vi "motortestMeng3.vi"() -> ()   [LabVIEW 2014]
uses:
  <vilib>/Utility/inputDevices.llb/joystickAcquire.vi
  <vilib>/Utility/inputDevices.llb/closeJoystick.vi
panel:
  in  "fRelDist":sgl
  in  "MG17Motor":refnum<k7>(container)
  out "Numeric":i32
  out "pfPosition":sgl
  in  "stop 2":bool
  in  "MG17Motor 2":refnum<k7>(container)
  out "button info":T1
  out "axis info":T2
  in  "stop":bool
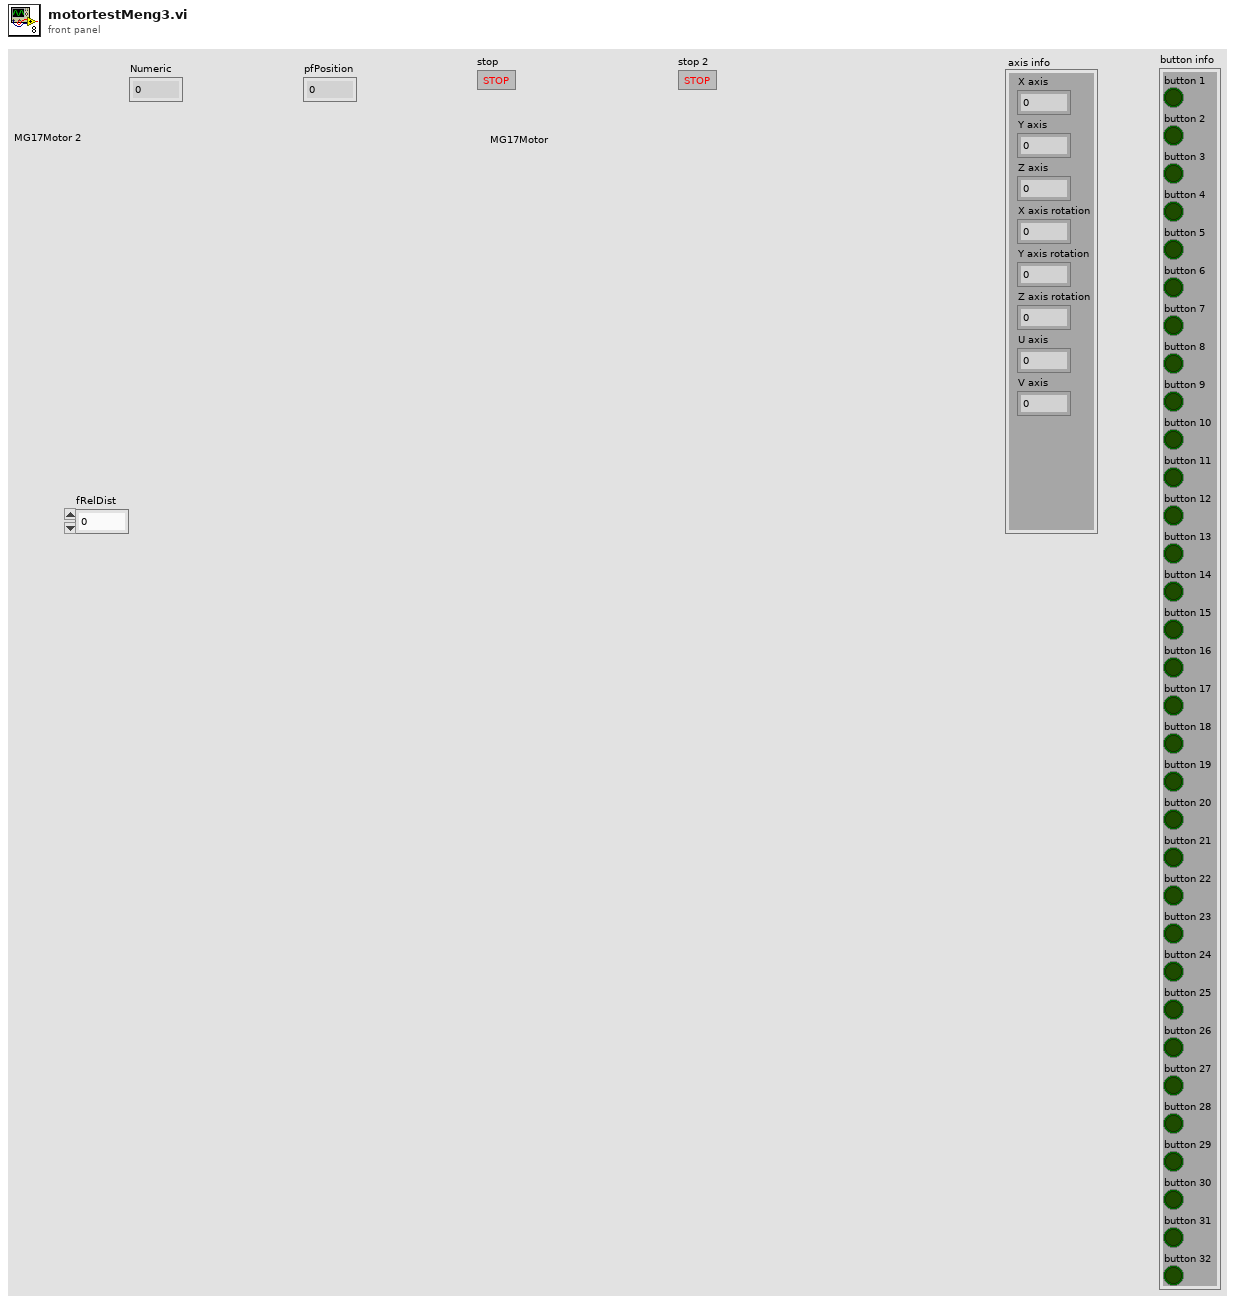
[diagram p1: front panel]
types:
  T1 = cluster{"button 1":bool, "button 2":bool, "button 3":bool, "button 4":bool, "button 5":bool, "button 6":bool, "button 7":bool, "button 8":bool, "button 9":bool, "button 10":bool, "button 11":bool, "button 12":bool, "button 13":bool, "button 14":bool, "button 15":bool, "button 16":bool, "button 17":bool, "button 18":bool, "button 19":bool, "button 20":bool, "button 21":bool, "button 22":bool, "button 23":bool, "button 24":bool, "button 25":bool, "button 26":bool, "button 27":bool, "button 28":bool, "button 29":bool, "button 30":bool, "button 31":bool, "button 32":bool}
  T2 = cluster{"X axis":i32, "Y axis":i32, "Z axis":i32, "X axis rotation":i32, "Y axis rotation":i32, "Z axis rotation":i32, "U axis":i32, "V axis":i32}
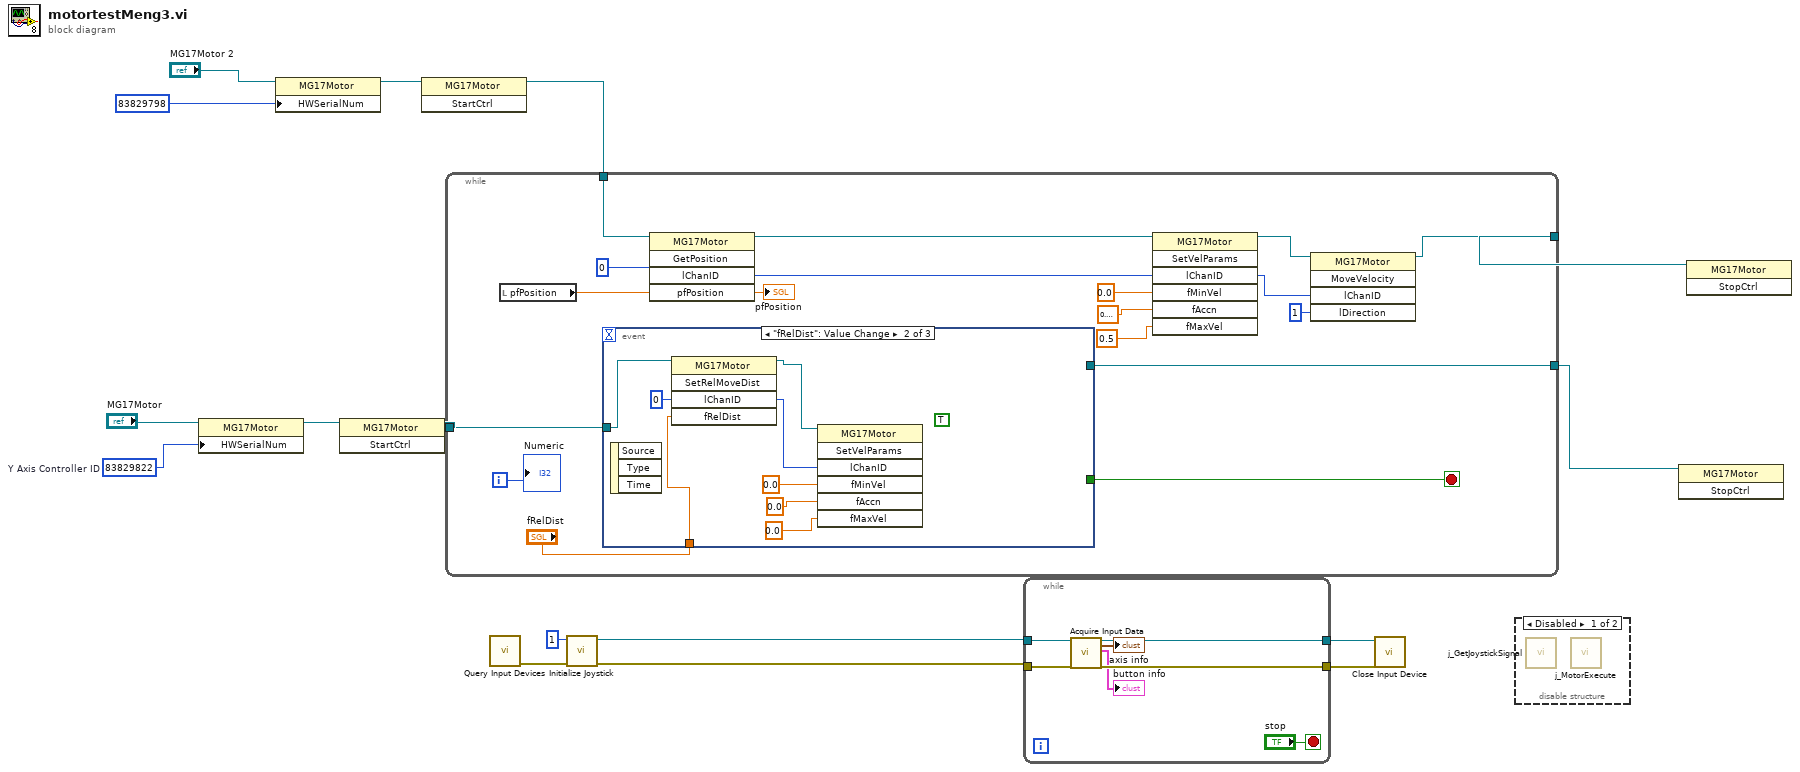
[diagram p0: block diagram]
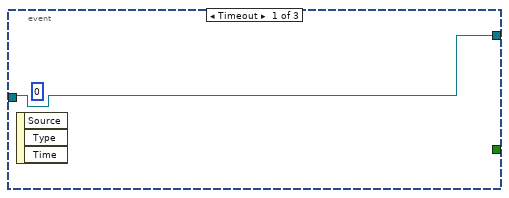
[diagram p3: hidden frame]
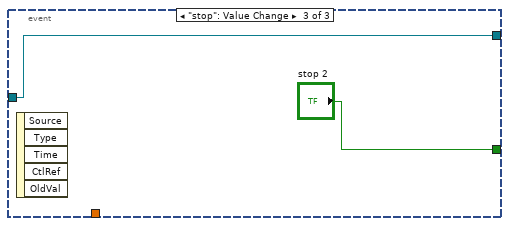
[diagram p4: hidden frame]
diagram:
  w5 = 83829822  # Y Axis Controller ID
  n1 = property class="MG17Motor"(reference="MG17Motor", "HWSerialNum"=w5) -> (reference out=w3:refnum<k7>)  [unwired: 1 in, 1 out]
  n2 = property class="MG17Motor"(reference="MG17Motor 2", "HWSerialNum"=83829798 ("Controller ID")) -> (reference out=w7:refnum<k7>)  [unwired: 1 in, 1 out]
  n3 = invoke class="MG17Motor" method="StartCtrl"(reference=w3) -> (reference out=w2:refnum<k7>)  [unwired: 2 in, 2 out]
  n4 = invoke class="MG17Motor" method="StartCtrl"(reference=w7) -> (reference out=w6:refnum<k7>)  [unwired: 2 in, 2 out]
  n5 = while {
    tunnel: [w28] -> w10
    tunnel: w6 -> [w33]
    tunnel: w2 -> [w20]
    tunnel: [w18] -> w1
    i -> [w34]
    stop <- w17 stop-if-true
    n6 = local read "pfPosition"() -> (w30:sgl)
    n7 = event shown="[1] \"fRelDist\": Value Change" {
      selector: _ -> [_ _ _]
      dyn-events: _ -> [_ _ _]
      timeout: _ -> [_ _ _]
      tunnel: "fRelDist" -> [_ w42 _]
      tunnel: w20 -> [w35 w43 w44]
      tunnel: [w35 _ w44] -> w18
      tunnel: [_ _ "stop 2"] -> w17
      event Timeout {
        (unwired) 0 ("lChanID")
        n8 = event-data() -> ()  [unwired: 1 in, 3 out]
      }
      event "fRelDist": Value Change {
        (unwired) TRUE ("bWait")
        n9 = event-data() -> ()  [unwired: 1 in, 3 out]
        n10 = invoke class="MG17Motor" method="SetRelMoveDist"(reference=w43, "lChanID"=0, "fRelDist"=w42) -> (reference out=w37:refnum<k7>, "lChanID"=w36:i32)  [unwired: 2 in, 3 out]
        n11 = invoke class="MG17Motor" method="SetVelParams"(reference=w37, "lChanID"=w36, "fMinVel"=sgl 0.0, "fAccn"=sgl 0.0 ("fMinVel"), "fMaxVel"=sgl 0.0 ("fMinVel")) -> ()  [unwired: 2 in, 7 out]
      }
      event "stop": Value Change {
        n12 = event-data() -> ()  [unwired: 1 in, 5 out]
      }
    }
    n13 = invoke class="MG17Motor" method="GetPosition"(reference=w33, "lChanID"=0, "pfPosition"=w30) -> (reference out=w22:refnum<k7>, "lChanID"=w27:i32, "pfPosition"=→"pfPosition":sgl)  [unwired: 2 in, 2 out]
    n14 = invoke class="MG17Motor" method="SetVelParams"(reference=w22, "lChanID"=w27, "fMinVel"=sgl 0.0, "fAccn"=sgl 0.3 ("fMinVel"), "fMaxVel"=sgl 0.5 ("fMinVel")) -> (reference out=w29:refnum<k7>, "lChanID"=w26:i32)  [unwired: 2 in, 5 out]
    n15 = invoke class="MG17Motor" method="MoveVelocity"(reference=w29, "lChanID"=w26, "lDirection"=1) -> (reference out=w28:refnum<k7>)  [unwired: 2 in, 4 out]
    "Numeric" <- w34
  }
  n16 = call <vilib>:"Query Input Devices.vi"() -> ("error out"=w15:errorcluster)  [unwired: 8 in, 3 out]
  n17 = call <vilib>:"Initialize Joystick.vi"("error in (no error)"=w15, "device index"=1) -> ("error out"=w13:errorcluster, "device ID"=w14:refnum<k1>)  [unwired: 8 in]
  n18 = while {
    tunnel: w14 -> [w52]
    tunnel: [w50] -> w12
    tunnel: w13 -> [w51]
    tunnel: [w49] -> w11
    stop <- "stop" stop-if-true
    n19 = call-poly <vilib>:"Acquire Input Data.vi"("device ID"=w52, "error in (no error)"=w51) -> ("device ID 2"=w50:refnum<k1>, "axis info"=→"axis info":T2, "button info"=→"button info":T1, "error out"=w49:errorcluster)  [unwired: 13 in, 1 out]
  }
  n20 = call-poly <vilib>:"Close Input Device.vi"("error in (no error)"=w11, "device ID"=w12) -> ()  [unwired: 8 in, 1 out]
  n21 = disable-structure shown="Disabled" {
    frame Disabled {
      n22 = call "j_GetJoystickSignal.vi"() -> ()  [unwired: 5 in, 5 out]
      n23 = call "j_MotorExecute.vi"() -> ()  [unwired: 6 in, 5 out]
    }
    frame Enabled {
    }
  }
  n24 = invoke class="MG17Motor" method="StopCtrl"(reference=w1) -> ()  [unwired: 2 in, 3 out]
  n25 = invoke class="MG17Motor" method="StopCtrl"(reference=w10) -> ()  [unwired: 2 in, 3 out]
